vi "initialize binary file.vi"(8 "error in":errorcluster, 10 "dictionary":T1, 11 "Byte Stream File in":refnum<file>) -> (0 "error out":errorcluster, 3 "Byte Stream File out":refnum<file>)   [LabVIEW 2013, in "Binary datalogger runtime.lvclass"]
uses:
  Binary datalogger runtime.lvclass
  <vilib>/NI/Tag Bus/dictionary/full data dictionary.ctl
  <vilib>/NI/Tag Bus/dictionary/data dictionary.lvclass
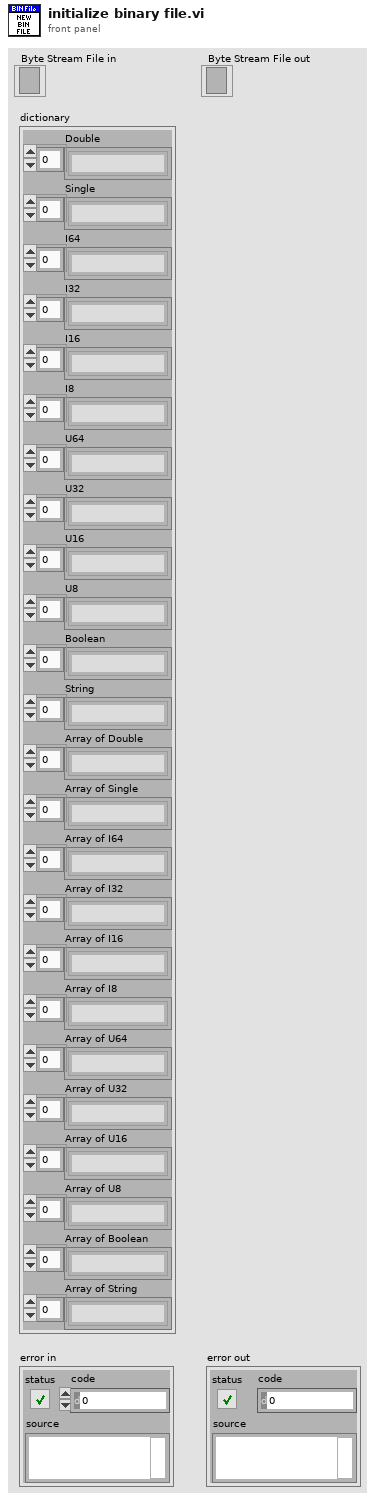
[diagram p1: front panel]
types:
  T1 = typedef "tag bus.lvlib/data dictionary.lvclass/full data dictionary.ctl" = cluster{"Double":string[], "Single":string[], "I64":string[], "I32":string[], "I16":string[], "I8":string[], "U64":string[], "U32":string[], "U16":string[], "U8":string[], "Boolean":string[], "String":string[], "Array of Double":string[], "Array of Single":string[], "Array of I64":string[], "Array of I32":string[], "Array of I16":string[], "Array of I8":string[], "Array of U64":string[], "Array of U32":string[], "Array of U16":string[], "Array of U8":string[], "Array of Boolean":string[], "Array of String":string[]}
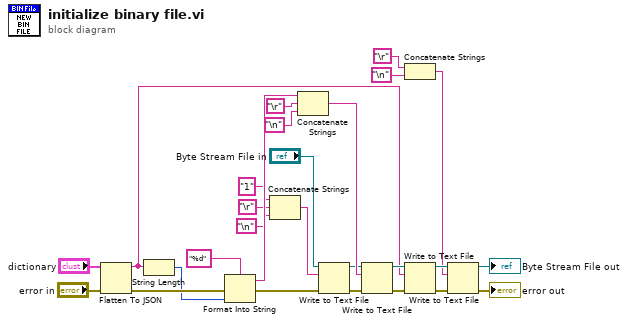
[diagram p0: block diagram]
diagram:
  n1 = Flatten To JSON(anything="dictionary", error in (no error)="error in") -> (JSON string=w20:string, 11:w24:errorcluster)  [unwired: 1 in]
  n2 = String Length(string=w20) -> (length=w23:i32)
  n3 = Format Into String(format string="%d", error in=w24, w23) -> (resulting string=w18:string, error out=w19:errorcluster)  [unwired: 1 in]
  n4 = Concatenate Strings("1" ("string"), "\r", "\n") -> (w1:string)
  n5 = Concatenate Strings(w18, "\r", "\n") -> (w15:string)
  n6 = Write to Text File(file (use dialog)="Byte Stream File in", text=w1, error in=w19) -> (refnum out=w5:refnum<file>, error out=w7:errorcluster)  [unwired: 1 in, 1 out]
  n7 = Write to Text File(file (use dialog)=w5, text=w15, error in=w7) -> (refnum out=w21:refnum<file>, error out=w27:errorcluster)  [unwired: 1 in, 1 out]
  n8 = Concatenate Strings("\r", "\n") -> (w8:string)
  n9 = Write to Text File(file (use dialog)=w21, text=w20, error in=w27) -> (refnum out=w14:refnum<file>, error out=w13:errorcluster)  [unwired: 1 in, 1 out]
  n10 = Write to Text File(file (use dialog)=w14, text=w8, error in=w13) -> (refnum out=→"Byte Stream File out":refnum<file>, error out=→"error out":errorcluster)  [unwired: 1 in, 1 out]
